vi "fitting_1d_pixel.vi"(6 "D sign":dbl, 7 "side velocity threshold":dbl, 8 "fitting axis":dbl, 9 "ratio_pixel2mil":dbl, 11 "array in":dbl[][](array[numeric])) -> (0 "D":ext[](array[numeric]), 2 "slope":dbl, 3 "fitting array":dbl[][](array[numeric]))   [LabVIEW 2017]
uses:
  <vilib>/Analysis/NI_AALPro.lvlib
panel:
  out "Array out 2":ext[](array[numeric])
  out "Array out":ext[](array[numeric])
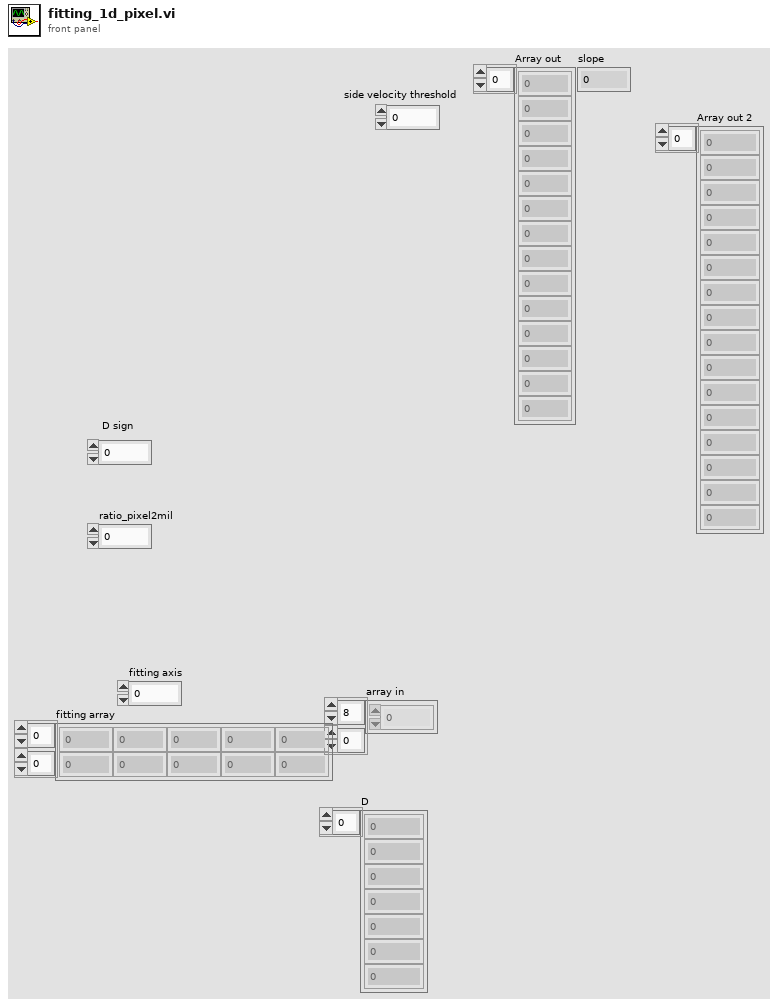
[diagram p1: front panel]
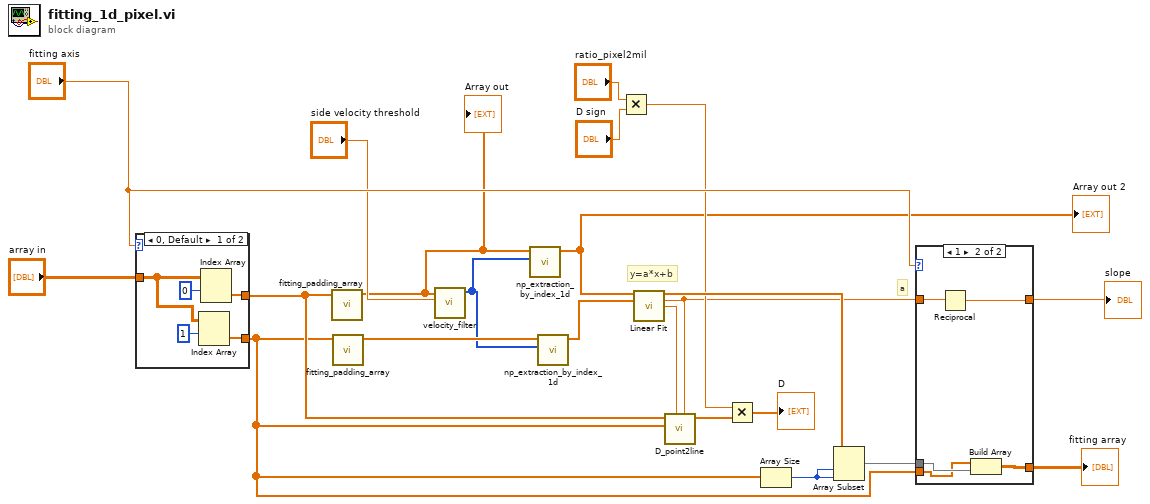
[diagram p0: block diagram]
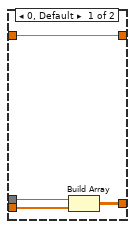
[diagram p2: hidden frame]
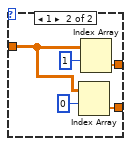
[diagram p3: hidden frame]
diagram:
  # "a"
  # "y=a*x+b"
  n1 = case shown="0, Default" "fitting axis" {
    tunnel: "array in" -> [w25 w30]
    tunnel: [w24 w29] -> w18
    tunnel: [w23 w28] -> w17
    frame 0, Default {
      n2 = Index Array(array=w25, index (row)=1) -> (element=w23:dbl[])  [unwired: 1 in]
      n3 = Index Array(array=w25, index (row)=0) -> (element=w24:dbl[])  [unwired: 1 in]
    }
    frame 1 {
      n4 = Index Array(array=w30, index (row)=0) -> (element=w28:dbl[])  [unwired: 1 in]
      n5 = Index Array(array=w30, index (row)=1) -> (element=w29:dbl[])  [unwired: 1 in]
    }
  }
  n6 = call "fitting_padding_array.vi"("array in"=w18) -> ("Array out"=w4:ext[])  [unwired: 10 in]
  "Array out" <- w4
  n7 = call "fitting_padding_array.vi"("array in"=w17) -> ("Array out"=w8:ext[])  [unwired: 10 in]
  n8 = call "velocity_filter.vi"("threshold"="side velocity threshold", "Array in"=w4) -> ("index"=w7:i32[])  [unwired: 9 in]
  n9 = call "np_extraction_by_index_1d.vi"("index array"=w7, "Array in"=w4) -> ("Array out"=w5:ext[])  [unwired: 9 in]
  "Array out 2" <- w5
  n10 = call "np_extraction_by_index_1d.vi"("index array"=w7, "Array in"=w8) -> ("Array out"=w6:ext[])  [unwired: 9 in]
  n11 = Multiply(x="ratio_pixel2mil", y="D sign") -> (x*y=w10:dbl)
  n12 = call <vilib>:"Linear Fit.vi"("Y"=w5, "X"=w6) -> ("Best Linear Fit"=w21:dbl[], "slope"=w3:dbl, "intercept"=w2:dbl)  [unwired: 9 in, 2 out]
  n13 = call "D_point2line.vi"("slope"=w3, "intercept"=w2, "X Array"=w17, "Y Array"=w18) -> ("D"=w15:ext[])  [unwired: 5 in, 2 out]
  n14 = Multiply(x=w10, y=w15) -> (x*y=→"D":ext[])
  n15 = Array Size(array=w17) -> (size(s)=w22:i32)
  n16 = Array Subset(array=w21, index=w22, length=w22) -> (w20:dbl[])
  n17 = case shown="1" "fitting axis" {
    tunnel: w20 -> [w36 w40]
    tunnel: w17 -> [w35 w39]
    tunnel: [w34 w41] -> w14
    tunnel: w3 -> [w33 w38]
    tunnel: [w33 w37] -> w1
    frame 0, Default {
      n18 = Build Array(w36, w35) -> (w34:dbl[][])
    }
    frame 1 {
      n19 = Reciprocal(x=w38) -> (1/x=w37:dbl)
      n20 = Build Array(w39, w40) -> (w41:dbl[][])
    }
  }
  "fitting array" <- w14
  "slope" <- w1
